vi "setMultiplot.vi"(6 "ScaleAdjust":dbl, 7 "OverallTitle":string, 9 "Cols":u8, 10 "Rows":u8, 11 "String in":string) -> (1 "nGraphs":i32, 3 "String out":string, 4 "command":string)   [LabVIEW 2012]
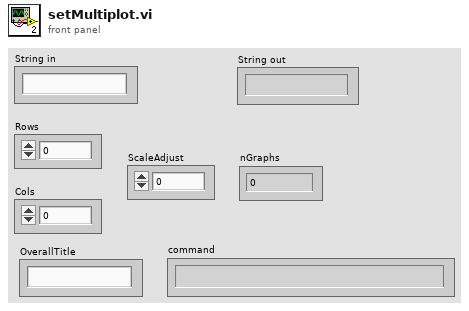
[diagram p1: front panel]
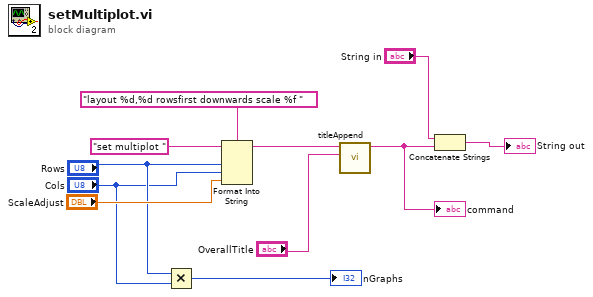
[diagram p0: block diagram]
diagram:
  n1 = Multiply(x="Rows", y="Cols") -> (x*y=→"nGraphs":u8)
  n2 = Format Into String(format string="layout %d,%d rowsfirst downwards scale %f ", initial string="set multiplot ", "Rows", "Cols", "ScaleAdjust") -> (resulting string=w9:string)  [unwired: 1 in, 1 out]
  n3 = call "titleAppend.vi"("Final Title"="OverallTitle", "String in"=w9) -> ("String out"=w1:string)  [unwired: 9 in]
  "command" <- w1
  n4 = Concatenate Strings("String in", w1) -> (→"String out":string)
